vi "ArmFF_New_ZeroGravity.vi"(9 "Ka":dbl, 10 "Kv":dbl, 11 "Ks":dbl) -> (3 "ARM_FF":T1 {"kCos" format="%13.5p"; "Ka" format="%13.5p"; "Kv" format="%13.5p"; "Ks" format="%13.5p"})   [LabVIEW 2019, in "Trajectory_Library.lvlib"]
doc: "Creates a new ArmFeedforward data cluster with the specified gains. Acceleration gain is defaulted to zero. Units of the gain values will dictate units of the computed feedforward.\n\nThis set of subVIs computes feedforward outputs for a simple arm (modeled as a motor acting against the force of gravity on a beam suspended at an angle).\n\nInputs: \n - ks -- The static gain.\n - kv -- The velocity gain.\n - ka -- The acceleration gain.\n - kcos -- The gravity gain.\n\nOutputs:\n - ArmFF -- The initialized ArmFF data cluster"
uses:
  Trajectory_Library.lvlib
  TypeDef/ARM_FF.ctl
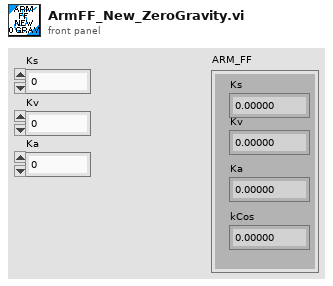
[diagram p1: front panel]
types:
  T1 = typedef "Trajectory_Library.lvlib/ARM_FF.ctl" = cluster{"Ks":dbl, "Kv":dbl, "Ka":dbl, "kCos":dbl}
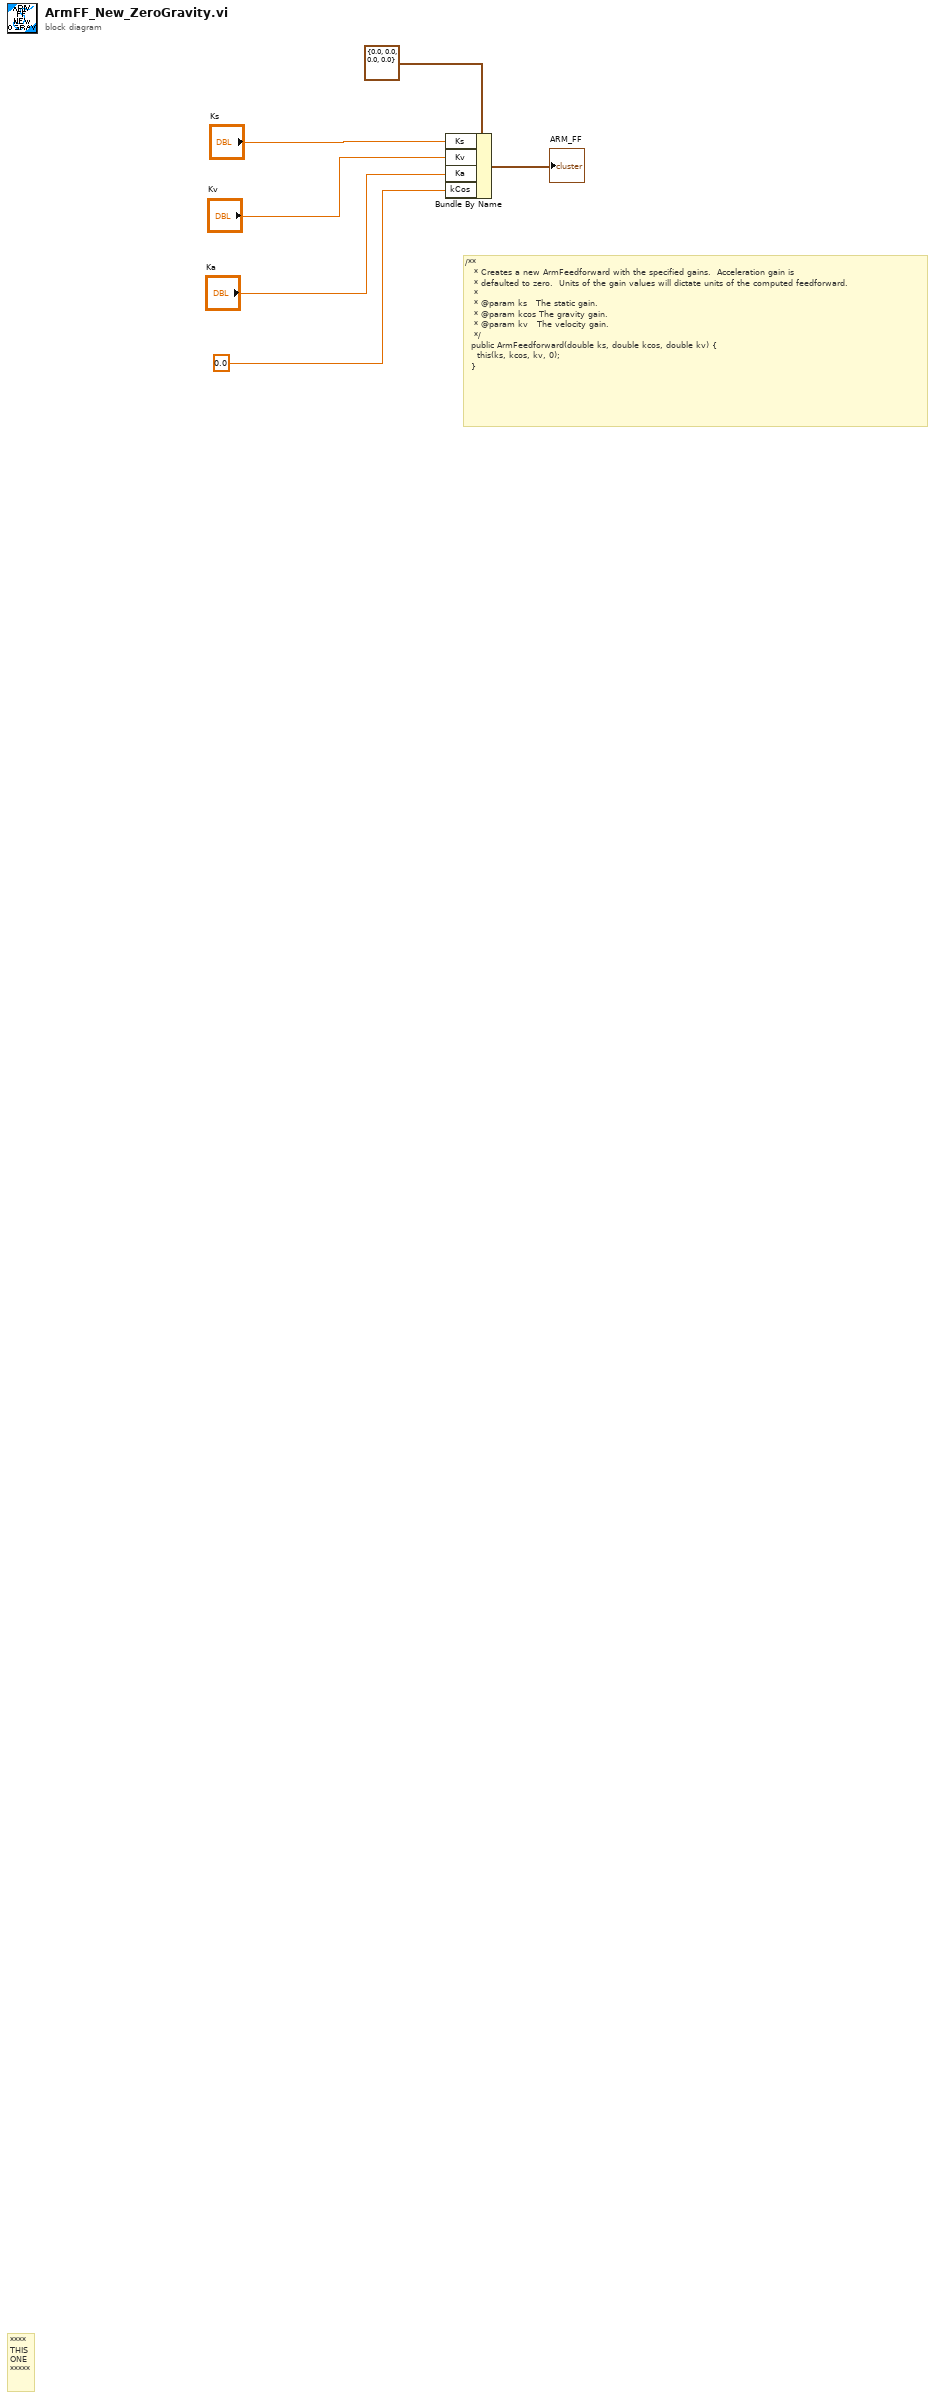
[diagram p0: block diagram]
diagram:
  # "/**\n   * Creates a new ArmFeedforward with the specified gains.  Acceleration gain is\n   * defaulted to zero.  Units of the gain values will dictate units of the computed feedforward.\n   *\n   * @param ks   The static gain.\n   * @param kcos The gravity gain.\n   * @param kv   The velocity gain.\n   */\n  public ArmFeedforward(double ks, double kcos, double kv) {\n    this(ks, kcos, kv, 0);\n  }"
  # "****\nTHIS\nONE\n*****"
  n1 = Bundle By Name(cluster=T1 {"Ks"=0.0, "Kv"=0.0, "Ka"=0.0, "kCos"=0.0} ("ARM_FF"), "Ks"="Ks", "Kv"="Kv", "Ka"="Ka", "kCos"=0.0) -> (→"ARM_FF":T1)
